vi "Goto P simples.vi"(6 "P":dbl, 8 "Theta":dbl, 9 "Y":dbl, 10 "X":dbl) -> (1 "w":dbl, 2 "Vy":dbl, 3 "Vx":dbl)   [LabVIEW 2016]
uses:
  <vilib>/Analysis/coordinate.llb/2D Cartesian Coordinate Rotation (Scalar).vi
  <vilib>/Analysis/NI_AALPro.lvlib
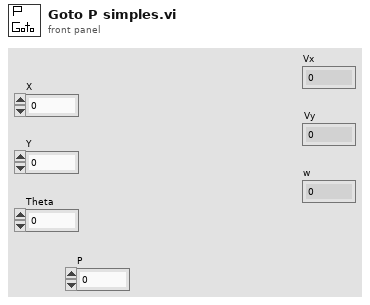
[diagram p1: front panel]
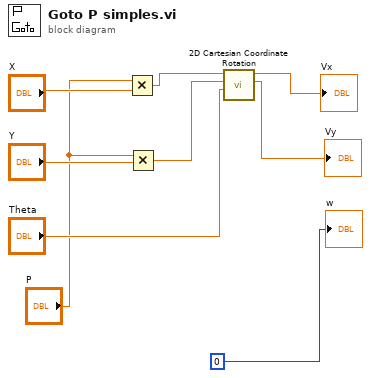
[diagram p0: block diagram]
diagram:
  n1 = Multiply(x="P", y="X") -> (x*y=w7:dbl)
  n2 = Multiply(x="P", y="Y") -> (x*y=w5:dbl)
  n3 = call-poly <vilib>:"2D Cartesian Coordinate Rotation.vi"("theta"="Theta", "y"=w5, "x"=w7) -> ("y out"=→"Vy":dbl, "x out"=→"Vx":dbl)  [unwired: 6 in, 1 out]
  "w" <- 0
